vi "Add Automation reference.vi"(8 "error in":errorcluster, 10 "Automation":variant, 11 "Fault Handler in":refnum<class "Fault Handler.lvclass">) -> (0 "error out":errorcluster, 3 "Fault Handler out":refnum<class "Fault Handler.lvclass">)   [LabVIEW 2019, in "Fault Handler.lvlib" / "Fault Handler.lvclass"]
doc: "<b>Add Automation Reference</b>\n\nThis routine take variant data (expected to be a TestStand Sequence Context reference) and writes the reference to private data."
uses:
  Project/Fault Handler.lvclass
  Project/Fault Handler.lvclass/Fault Handler.ctl
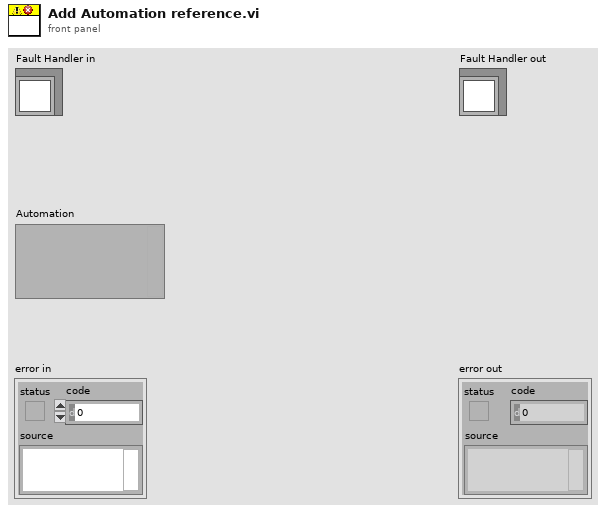
[diagram p1: front panel]
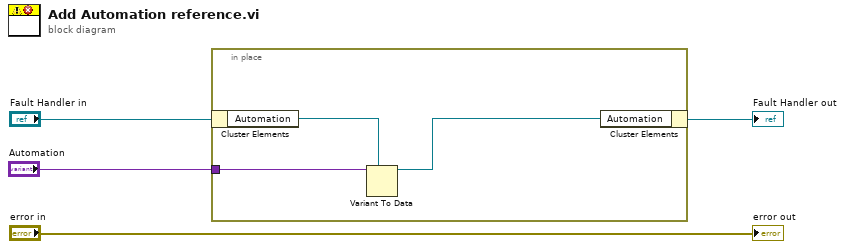
[diagram p0: block diagram]
diagram:
  n1 = in-place {
    in-place-border: "Automation" -> [w7]
    n2 = in-place-cluster #1("Fault Handler in") -> ("Automation"=w6:refnum<k7>)
    n3 = Variant To Data(type=w6, Variant=w7) -> (data=w5:refnum<k7>)  [unwired: 1 in, 1 out]
    n4 = in-place-cluster #1("Automation"=w5) -> (→"Fault Handler out":refnum<class "Fault Handler.lvclass">)
  }
  "error out" <- "error in"
